vi "Lookup Chart Reference.vi"(4 "Error In":errorcluster, 7 "Plugin Name":T1) -> (0 "Error Out":errorcluster, 3 "Reference Out":refnum<vi>)   [LabVIEW 2015, in "Plugin Chart References.lvlib"]
uses:
  Plugin Chart References.lvlib
  _libraries/Startup Processes/_typedefs/Subpanel Names.ctl
  _libraries/Startup Processes/Startup Processes.lvlib
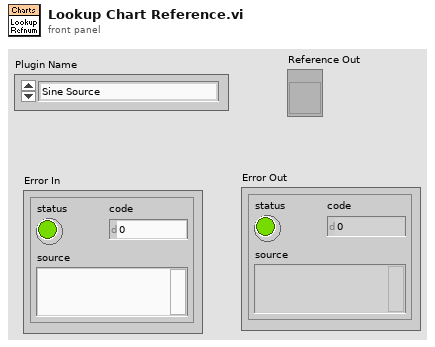
[diagram p1: front panel]
types:
  T1 = typedef "Startup Processes.lvlib/Subpanel Names.ctl" = enum16{"Sine Source", "Ramp Source", "Hen House TC", "Dog House TC", "Out House TC"}
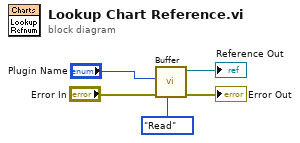
[diagram p0: block diagram]
diagram:
  n1 = call "Buffer.vi"("Function"=enum16{"Read", "Insert"}."Read", "Error In"="Error In", "Plugin Name"="Plugin Name") -> ("Error Out"=→"Error Out":errorcluster, "Reference Out"=→"Reference Out":refnum<vi>)  [unwired: 4 in]
